vi "Calibrate Phase.vi"(8 "error in (no error)":errorcluster, 9 "Boolean":bool, 10 "Results":T1 {"Results (Dictionary)"."value" format="%#_6p"}, 11 "Instrument.DAQ in":refnum<class "Instrument.DAQ.lvclass">) -> (0 "error out":errorcluster, 3 "Instrument.DAQ out":refnum<class "Instrument.DAQ.lvclass">)   [LabVIEW 2019, in "Instrument.Lockin.lvlib" / "Instrument.DAQ.lvclass"]
uses:
  Instrument.DAQ.lvclass
  Typedefs/Results--Cluster.ctl
  Instrument.Lockin/Typedefs/Results Type--Enum.ctl
  Instrument.DAQ.lvclass/Instrument.DAQ.ctl
  Instrument.Lockin/Instrument.Lockin.lvclass
  <vilib>/addons/control/pid/pid.llb/PID Control Input Filter (DBL).vi
panel:
  in  "Input/Ouput Map":cluster{"output":i32, "input":i32}[](array[cluster])
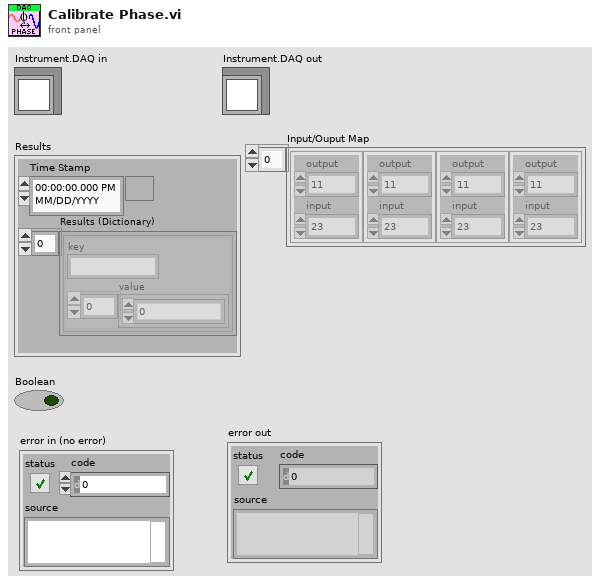
[diagram p1: front panel]
types:
  T1 = typedef "Instrument.Lockin.lvlib/Instrument.DAQ.lvclass/Results--Cluster.ctl" = cluster{"Time Stamp":timestamp, "Results (Dictionary)":cluster{"key":string, "value":dbl[]}[]}
  T2 = typedef "Instrument.Lockin.lvlib/Instrument.Lockin.lvclass/Results Type--Enum.ctl" = enum16{"X", "Y", "R", "Theta", "Mean"}
  T3 = typedef "Instrument.Lockin.lvlib/Instrument.DAQ.lvclass/AO.Channel--Cluster--Array.ctl" = T4[]
  T4 = typedef "Instrument.Lockin.lvlib/Instrument.DAQ.lvclass/AO.Channel--Cluster.ctl" = cluster{"Enable?":bool, "Channel":i32, "Amplitude":dbl, "Offset":dbl, "Frequency":dbl, "Phase":dbl, "Function":T5, "Sweeping?":bool, "Limit AC":bool, "Limit DC?":bool, "Duty Cycle":bool}
  T5 = typedef "Instrument.Lockin.lvlib/Instrument.DAQ.lvclass/AO.Channel.Function--Enum.ctl" = enum16{"sine", "square", "triangle", "saw"}
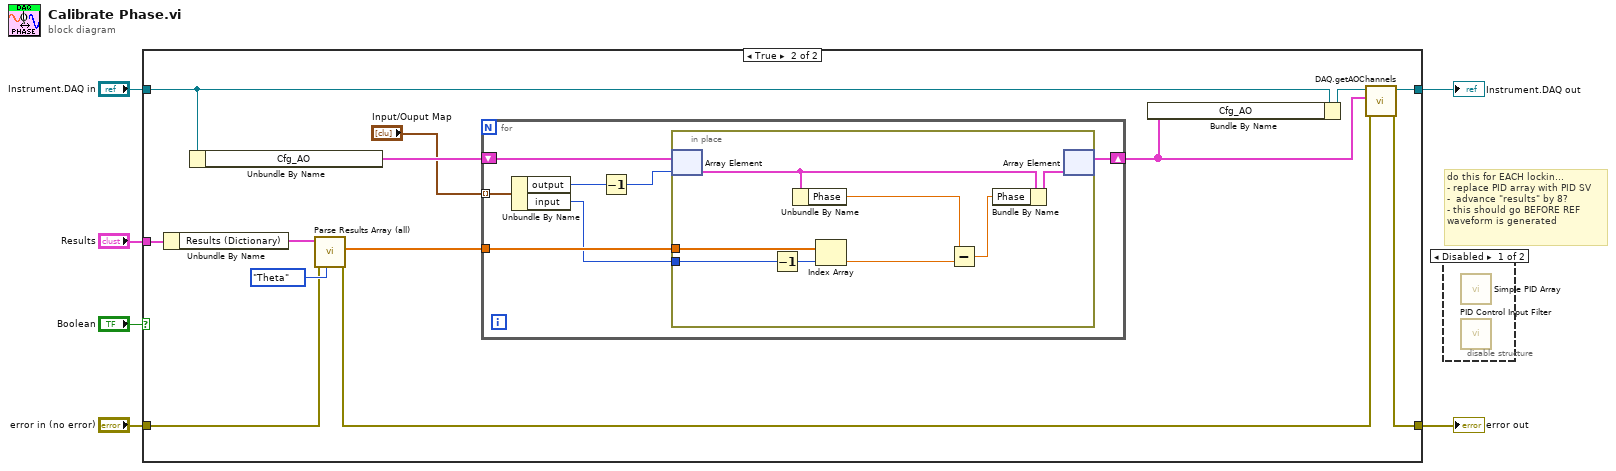
[diagram p0: block diagram]
diagram:
  # "do this for EACH lockin...\n- replace PID array with PID SV\n-  advance \"results\" by 8?\n- this should go BEFORE REF\nwaveform is generated"
  n1 = case shown="True" "Boolean" {
    tunnel: "Instrument.DAQ in" -> [w8 w9]
    tunnel: "Results" -> [_ w21]
    tunnel: "error in (no error)" -> [w7 w10]
    tunnel: [w8 w20] -> w3
    tunnel: [w7 w13] -> w2
    frame False {
    }
    frame True {
      n2 = Unbundle By Name(w21) -> ("Results (Dictionary)"=w19:cluster{"key":string, "value":dbl[]}[])
      n3 = Unbundle By Name(w9) -> ("Cfg_AO"=w15:T3)
      n4 = call "Parse Results Array (all).vi"("Type"=Results_Type--Enum."Theta", "error in (no error)"=w10, "Results (Dictionary)"=w19) -> ("error out"=w16:errorcluster, "Data"=w12:dbl[])  [unwired: 5 in, 2 out]
      n5 = for {
        tunnel: "Input/Ouput Map" -> [w28] mode=indexing
        shift-right: [w22] -> w11
        shift-left: w15 -> [w25]
        tunnel: w12 -> [w27]
        n6 = Unbundle By Name(w28) -> ("output"=w24:i32, "input"=w26:i32)
        n7 = Decrement(x=w24) -> (x-1=w23:i32)
        n8 = in-place {
          in-place-border: w27 -> [w29]
          in-place-border: w26 -> [w32]
          n9 = in-place-array #1(w25, w23) -> (w30:T4)
          n10 = Decrement(x=w32) -> (x-1=w36:i32)
          n11 = Unbundle By Name(w30) -> ("Phase"=w35:dbl)
          n12 = Index Array(array=w29, index=w36) -> (element=w34:dbl)
          n13 = Subtract(x=w35, y=w34) -> (x-y=w33:dbl)
          n14 = Bundle By Name(cluster=w30, "Phase"=w33) -> (w31:T4)
          n15 = in-place-array #1(w31) -> (w22:T3)  [unwired: 1 out]
        }
      }
      n16 = Bundle By Name(cluster=w9, "Cfg_AO"=w11) -> (w17:refnum<class "Instrument.DAQ.lvclass">)
      n17 = call "DAQ.getAOChannels.vi"("error in (no error)"=w16, "Channels: AO"=w11, "Instrument.DAQ"=w17) -> ("error out"=w13:errorcluster, "Instrument.DAQ out"=w20:refnum<class "Instrument.DAQ.lvclass">)  [unwired: 7 in]
    }
  }
  "Instrument.DAQ out" <- w3
  "error out" <- w2
  n18 = disable-structure shown="Disabled" {
    frame Disabled {
      n19 = call "Simple PID Array.vi"() -> ()  [unwired: 11 in, 1 out]
      n20 = call-poly <vilib>:"PID Control Input Filter.vi"() -> ()  [unwired: 5 in, 1 out]
    }
    frame Enabled {
    }
  }
